vi "Update Dummy Structure Table.vi"(8 "error in":errorcluster) -> (0 "error out":errorcluster)   [LabVIEW 2020, in "Scripts.lvlib"]
uses:
  Quick Drop/_Enclose in Structure/Get Dummy Structure Reference.vi
  Scripts.lvlib
  Quick Drop/_Enclose in Structure/Enclose in Structure.lvlib
  <vilib>/Utility/traverseref.llb/TRef TravTarget.ctl
  Quick Drop/_Enclose in Structure/Structure Type.ctl
  <vilib>/Utility/Data Type/NI_Data Type.lvlib
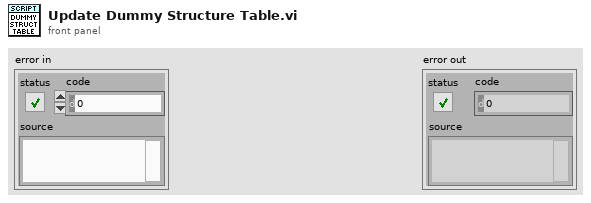
[diagram p1: front panel]
types:
  T1 = typedef "TRef TravTarget.ctl" = enum16{"FP", "BD", "Other"}
  T2 = typedef "Enclose in Structure.lvlib/Structure Type.ctl" = enum16{"<Invalid>", "For Loop", "While Loop", "Timed Loop", "Timed Sequence", "Case Structure", "Event Structure", "In Place Element Structure", "Flat Sequence", "Diagram Disable Structure", "Conditional Disable Structure", "Type Specialization Structure"}
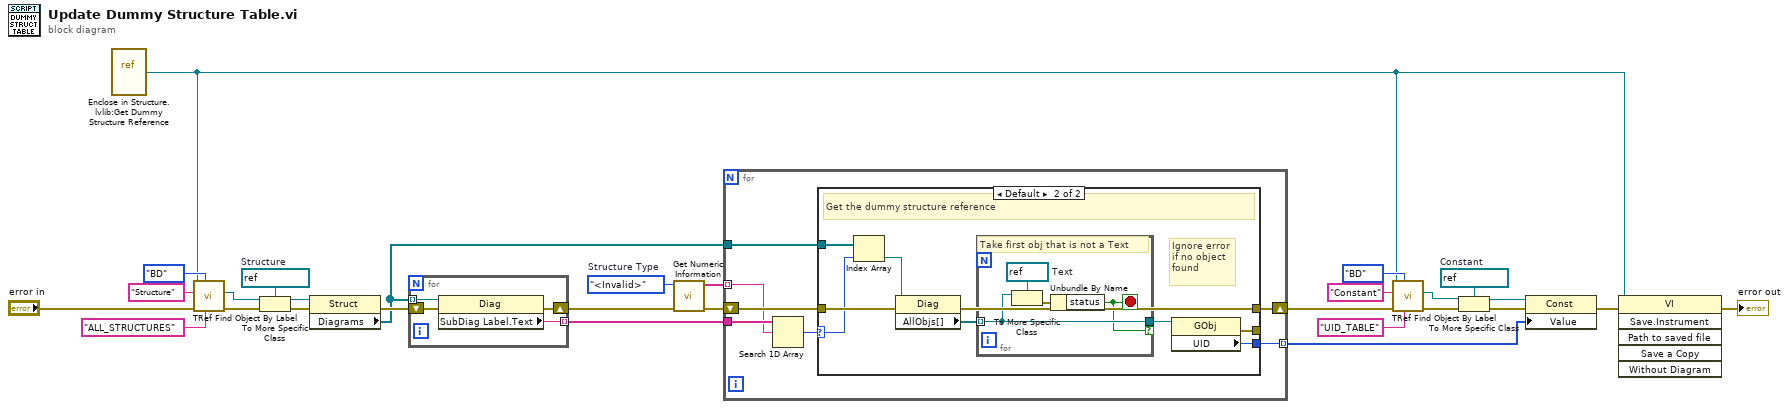
[diagram p0: block diagram]
diagram:
  w12 = refnum<vi> refnum  # Constant
  w23 = refnum<vi> refnum  # Structure
  w25 = Structure_Type."<Invalid>"  # Structure Type
  n1 = vi-ref "Enclose in Structure.lvlib:Get Dummy Structure Reference.vi"() -> (w1:refnum<vi>)
  n2 = call <vilib>:"TRef Find Object By Label.vi"("Label"="ALL_STRUCTURES", "Traverse Target"=TRef_TravTarget."BD", "error in (no error)"="error in", "Class Name"="Structure", "VI Ref"=w1) -> ("error out"=w21:errorcluster, "Found Obj Ref"=w24:refnum<vi>)  [unwired: 3 in, 2 out]
  n3 = To More Specific Class(target class=w23, reference=w24, error in=w21) -> (specific class reference=w22:refnum<vi>, error out=w20:errorcluster)
  n4 = property class="Struct"(reference=w22, error in=w20) -> (error out=w19:errorcluster, "Diagrams"=w14:refnum<vi>[])  [unwired: 1 out]
  n5 = for {
    tunnel: w14 -> [w33] mode=indexing
    tunnel: [w32] -> w18 mode=indexing
    shift-right: [w30] -> w17
    shift-left: w19 -> [w31]
    n6 = property class="Diag"(reference=w33, error in=w31) -> (error out=w30:errorcluster, "SubDiag Label.Text"=w32:string)  [unwired: 1 out]
  }
  n7 = call <vilib>:"Get Numeric Information.vi"("error in (no error)"=w17, "variant"=w25) -> ("error out"=w16:errorcluster, "enum names"=w15:string[])  [unwired: 6 in, 2 out]
  n8 = for {
    tunnel: w18 -> [w39]
    tunnel: w15 -> [w38] mode=indexing
    tunnel: w14 -> [w35]
    shift-right: [w36] -> w7
    shift-left: w16 -> [w40]
    tunnel: [w34] -> w4 mode=indexing
    n9 = Search 1D Array(1D array=w39, element=w38) -> (index of element=w37:i32)  [unwired: 1 in]
    n10 = case shown="Default" w37 {
      selector: w37 -> [_ w42]
      tunnel: w40 -> [w41 w50]
      tunnel: [w41 w49] -> w36
      tunnel: w35 -> [_ w43]
      tunnel: [_ w48] -> _
      tunnel: [_ w47] -> w34
      frame -1 {
        # "No subdiagram label corresponds to this structure type"
      }
      frame Default {
        # "Ignore error if no object found"
        # "Get the dummy structure reference"
        n11 = Index Array(array=w43, index=w42) -> (element=w44:refnum<vi>)
        n12 = property class="Diag"(reference=w44, error in=w50) -> (error out=w49:errorcluster, "AllObjs[]"=w46:refnum<vi>[])  [unwired: 1 out]
        n13 = for {
          tunnel: w46 -> [w53] mode=indexing
          tunnel: [w53] -> w45 if=w51
          stop <- w51 stop-if-true
          w54 = refnum<vi> refnum  # Text
          # "Take first obj that is not a Text"
          n14 = To More Specific Class(target class=w54, reference=w53) -> (error out=w52:errorcluster)  [unwired: 1 in, 1 out]
          n15 = Unbundle By Name(w52) -> ("status"=w51:bool)
        }
        n16 = property class="GObj"(reference=w45) -> (error out=w48:errorcluster, "UID"=w47:i32)  [unwired: 1 in, 1 out]
      }
    }
  }
  n17 = call <vilib>:"TRef Find Object By Label.vi"("Label"="UID_TABLE", "Traverse Target"=TRef_TravTarget."BD", "error in (no error)"=w7, "Class Name"="Constant", "VI Ref"=w1) -> ("error out"=w13:errorcluster, "Found Obj Ref"=w11:refnum<vi>)  [unwired: 3 in, 2 out]
  n18 = To More Specific Class(target class=w12, reference=w11, error in=w13) -> (specific class reference=w5:refnum<vi>, error out=w6:errorcluster)
  n19 = property class="Const"(reference=w5, error in=w6, "Value"=w4) -> (error out=w3:errorcluster)  [unwired: 1 out]
  n20 = invoke class="VI" method="Save.Instrument"(reference=w1, error in=w3) -> (error out=→"error out":errorcluster)  [unwired: 4 in, 5 out]
